vi "Process.vi"(8 "error in":errorcluster, 11 "Example Instrument":refnum<class "Instrument.LN2.lvclass">) -> (0 "error out":errorcluster, 3 "Example Instrument out":refnum<class "Instrument.LN2.lvclass">)   [LabVIEW 2019, in "Instrument.LN2.lvclass"]
doc: "---------------------------------------------------------------\nJKI State Machine Objects™\nhttp://jki.net/state-machine-objects/\nCopyright (C) 2005-2015, JKI <info@jki.net>\nALL RIGHTS RESERVED"
uses:
  Instrument.LN2.lvclass
  C:/Program Files (x86)/National Instruments/LabVIEW 2019/vi.lib/JKI/JKI SMO/SMO/SMO.lvclass
  C:/Program Files (x86)/National Instruments/LabVIEW 2019/user.lib/LevyLab/Instrument Framework/SMOs/Instrument/Instrument.lvclass
  Typedefs/PrivateEvents--Instrument.MessageToProcess.ctl
  <userlib>/LevyLab/Instrument Framework/SMOs/RemoteControl/Typedefs/Message--Cluster.ctl
  Instrument.LN2.lvclass/Instrument.LN2.ctl
  <vilib>/JKI/JKI SMO/SMO/SMO.lvclass/SMO.ctl
  Typedefs/Instrument.LN2.getAll--Cluster.ctl
  <vilib>/JKI/JKI SMO/SMO/Private/ReftoDVR--SMO.vi
  <userlib>/LevyLab/Instrument Framework/Instrument Types/VSource/Instrument.VSource.lvclass
  <vilib>/JKI/JKI SMO/SMO/SMO.lvclass
  <userlib>/LevyLab/Instrument Framework/SMOs/Instrument/Instrument.lvclass
  <userlib>/LevyLab/Instrument Framework/SMOs/RemoteControl/RemoteControl.lvclass
panel:
  # "LN2 process:\ntalks to hw"
  # "For instructions on how to use the JKI State Machine Objects, examples and video tutorials, visit:\nhttp://jki.net/state-machine-objects/\n\nJKI State Machine Objects™\nhttp://jki.net/state-machine-objects/\nCopyright (C) 2005-2015, JKI <info@jki.net>\nALL RIGHTS RESERVED"
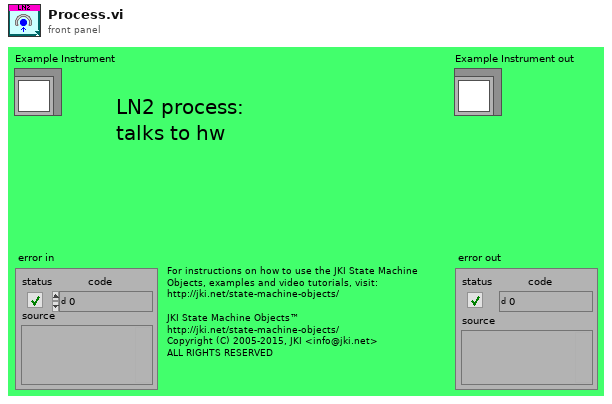
[diagram p1: front panel]
types:
  T1 = enum32{"invalid app kind", "Development System", "Run Time System", "Student Edition", "Embedded LabVIEW", "Evaluation", "Custom"}
  T2 = enum32{"Invalid", "Standard", "Closed", "Hidden", "Minimized", "Maximized"}
  T3 = enum32{"Bad", "Idle", "Run top level", "Running"}
  T4 = typedef "Instrument.LN2.lvclass/Instrument.LN2.getAll--Cluster.ctl" = cluster{"Net Weight(lbs)":dbl, "Level":dbl, "Status":string}
  T5 = typedef "RemoteControl.lvclass/Message--Cluster.ctl" = cluster{"Command":string, "Data":variant, "ID":string}
  T6 = typedef "Instrument.LN2.lvclass/PrivateEvents--Instrument.MessageToProcess.ctl" = cluster{"Message":T5}
  T7 = cluster{"Core":cluster{"Current VI Reference":refnum<vi>, "Close Panel on Exit?":bool, "Last Error":cluster{"error":errorcluster, "previous state":string, "remaining states":string}, "Shutdown?":bool}, "SelfRef":refnum<class "Instrument.LN2.lvclass">, "MessageToProcess":T6}
  T8 = cluster{"Current VI Reference":refnum<vi>, "Close Panel on Exit?":bool, "Last Error":cluster{"error":errorcluster, "previous state":string, "remaining states":string}, "Shutdown?":bool}
  T9 = typedef "SMO.lvclass/Protected Events.ctl" = cluster{"StopProcesses":refnum<user-event>, "AbortProcesses":refnum<user-event>, "Config Changed":refnum<user-event>, "Dependency":refnum<user-event>}
  T10 = typedef "Instrument.LN2.lvclass/PrivateEvents--Cluster.ctl" = cluster{"MessageToProcess":refnum<user-event>}
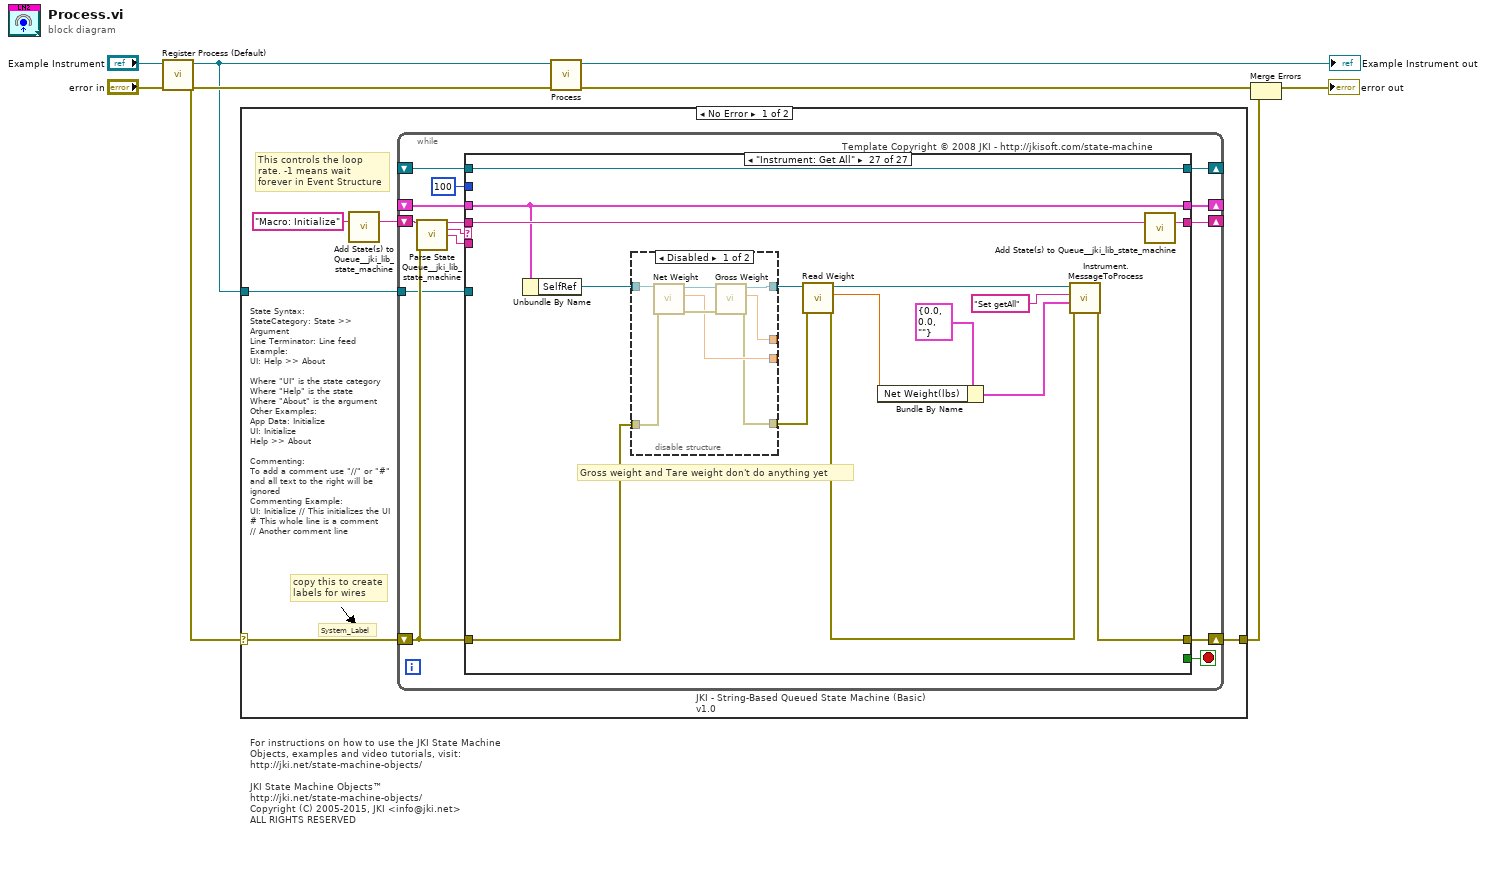
[diagram p0: block diagram]
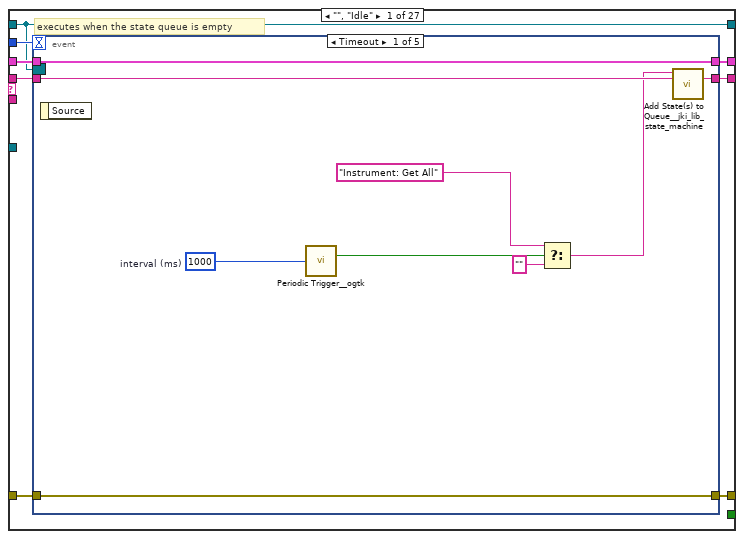
[diagram p2: hidden frame]
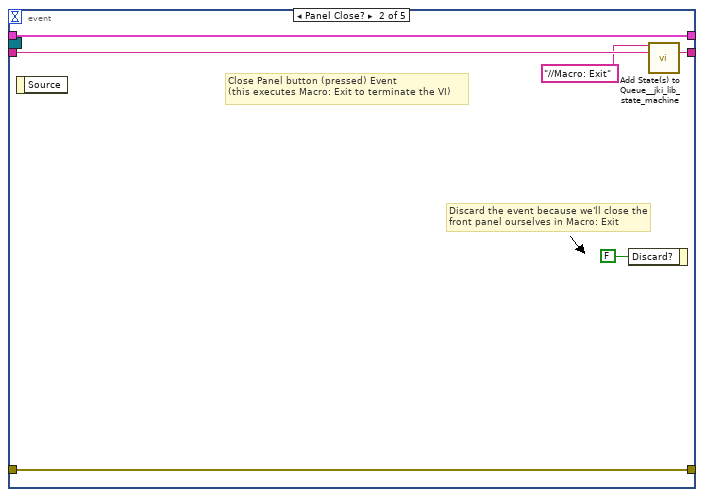
[diagram p3: hidden frame]
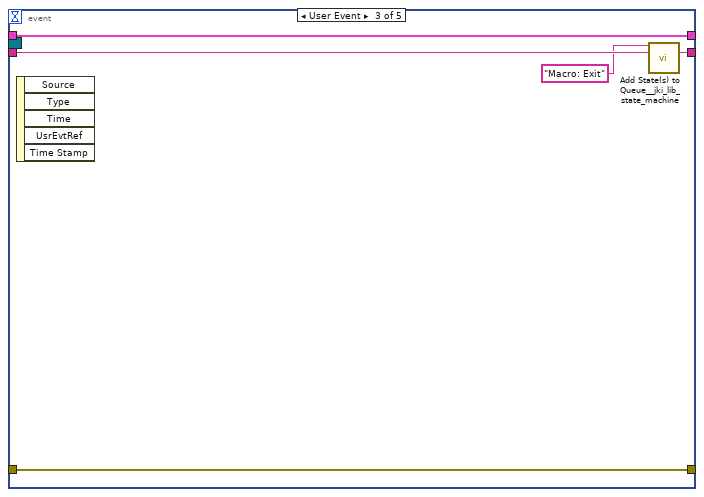
[diagram p4: hidden frame]
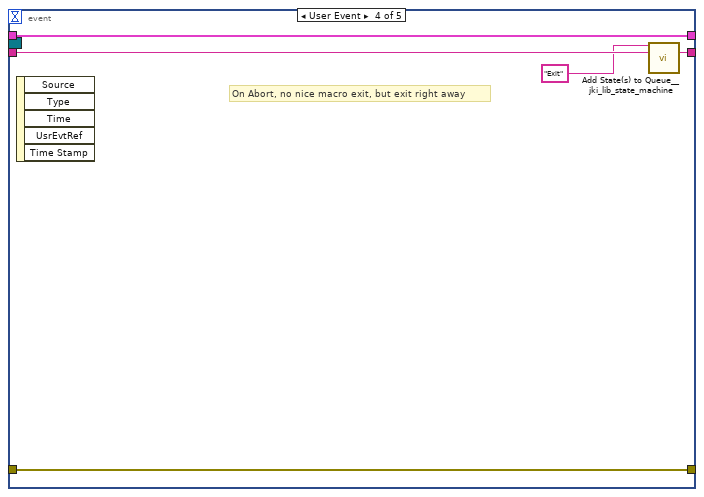
[diagram p5: hidden frame]
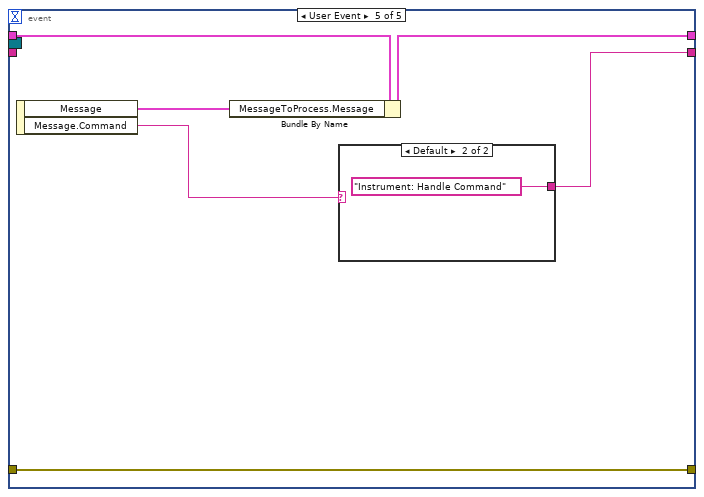
[diagram p6: hidden frame]
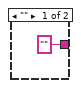
[diagram p7: hidden frame]
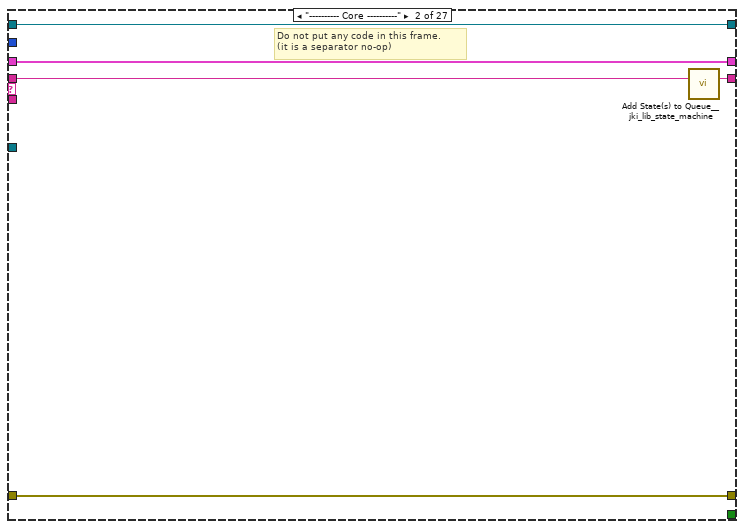
[diagram p8: hidden frame]
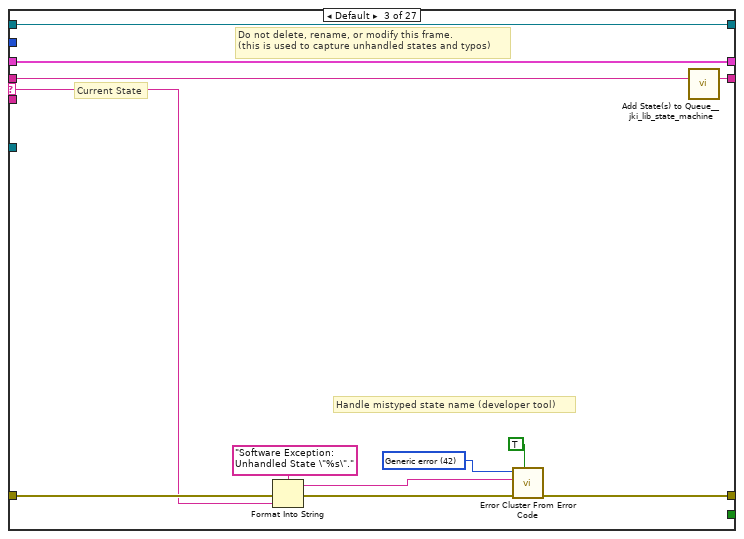
[diagram p9: hidden frame]
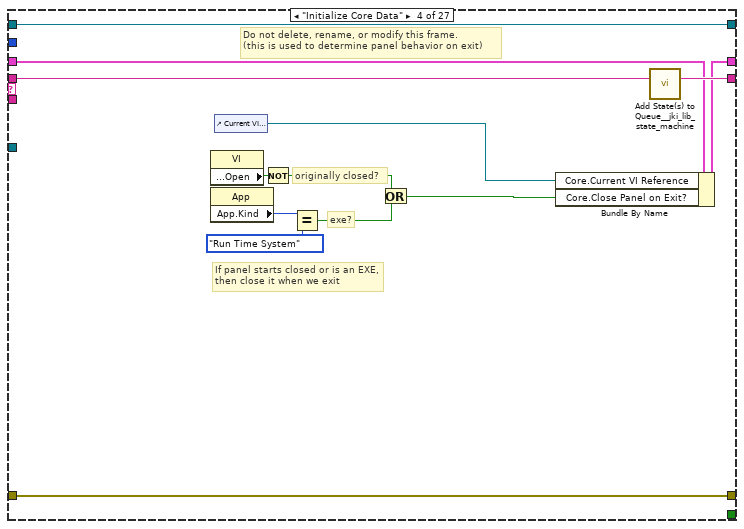
[diagram p10: hidden frame]
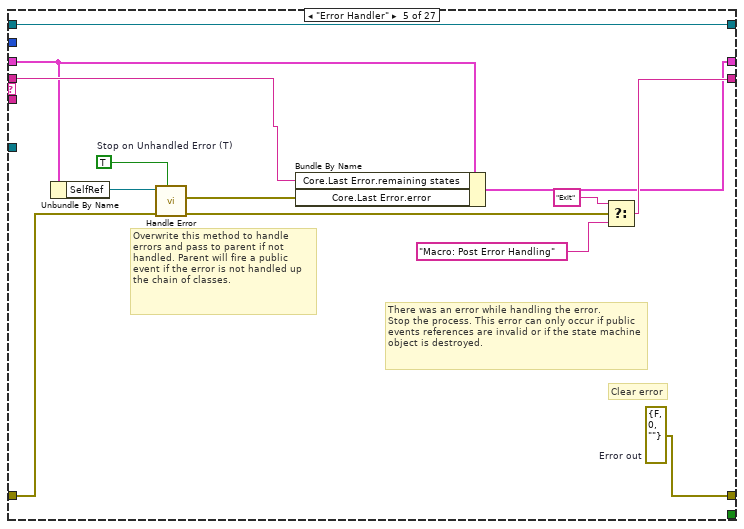
[diagram p11: hidden frame]
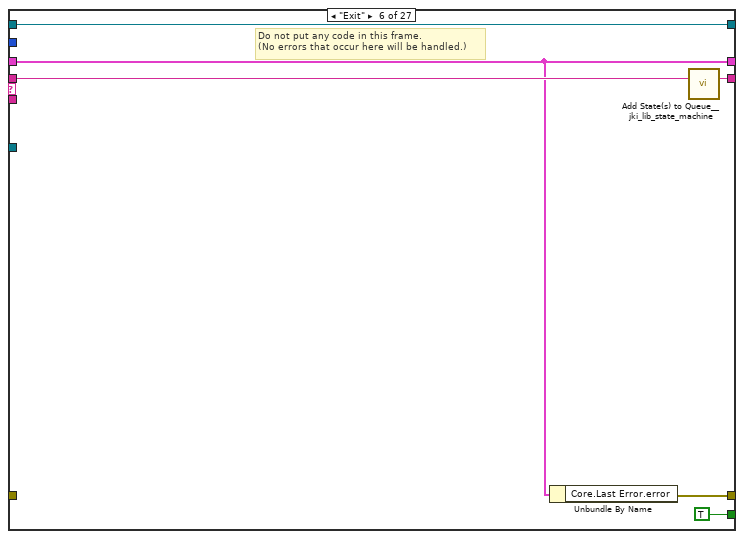
[diagram p12: hidden frame]
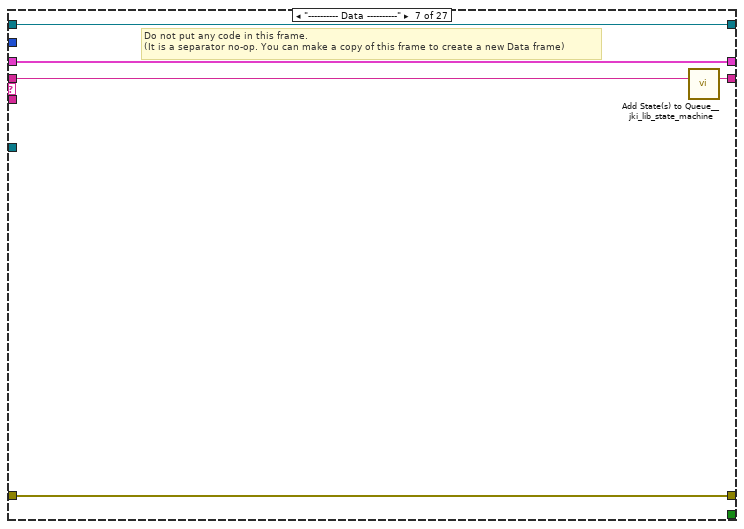
[diagram p13: hidden frame]
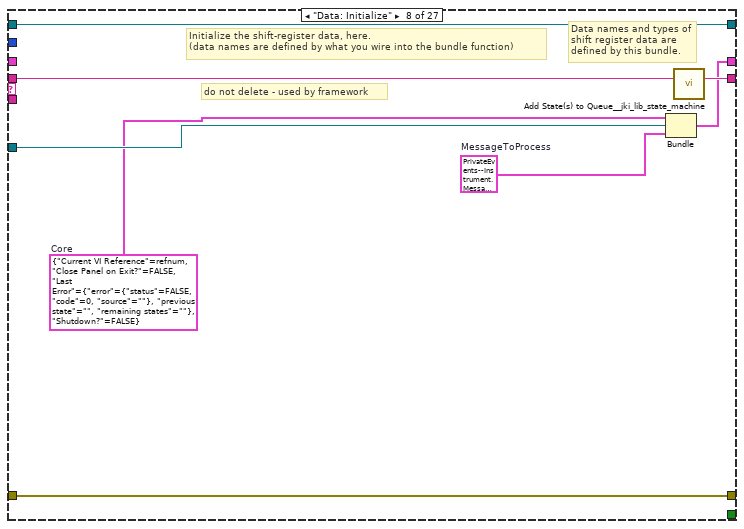
[diagram p14: hidden frame]
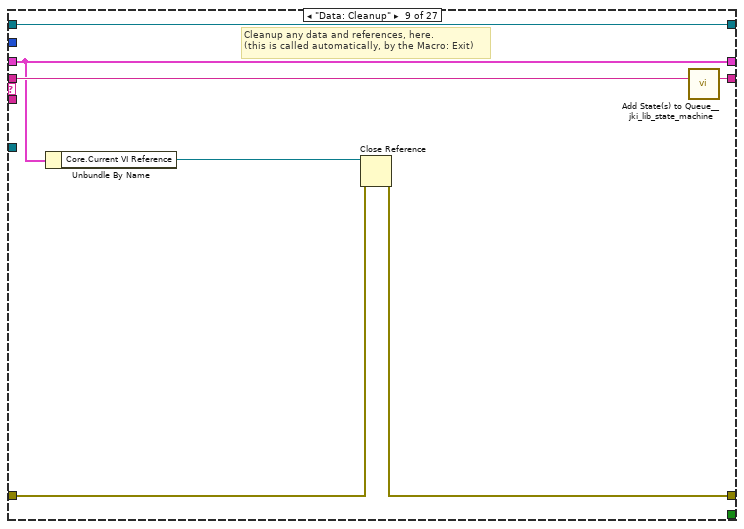
[diagram p15: hidden frame]
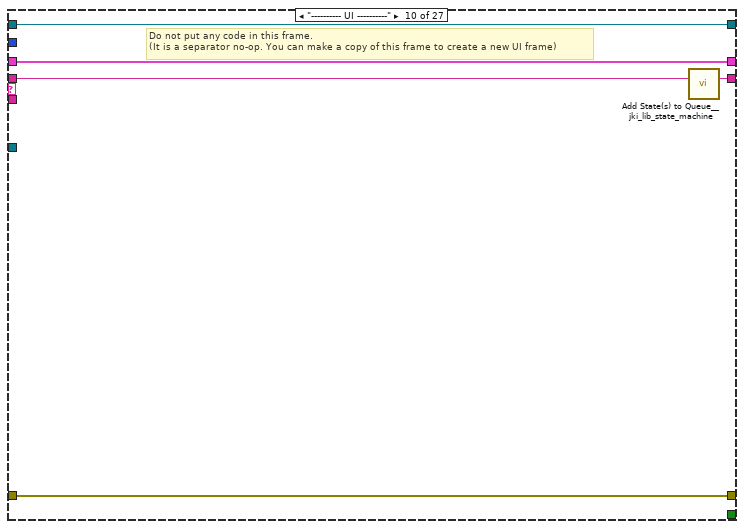
[diagram p16: hidden frame]
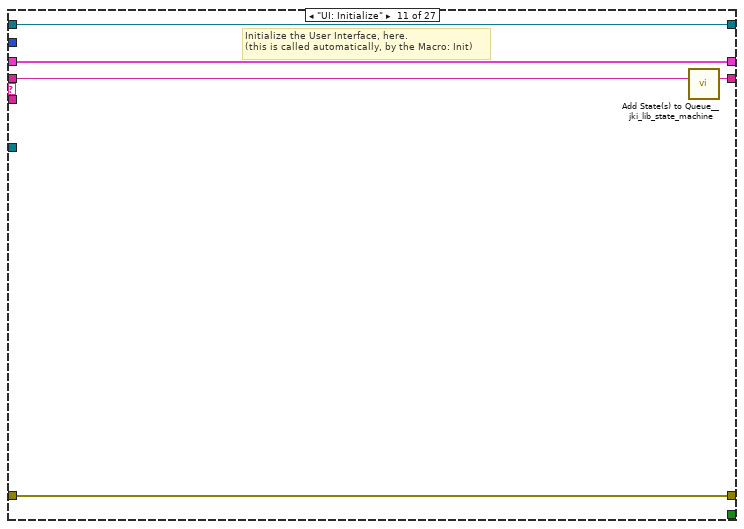
[diagram p17: hidden frame]
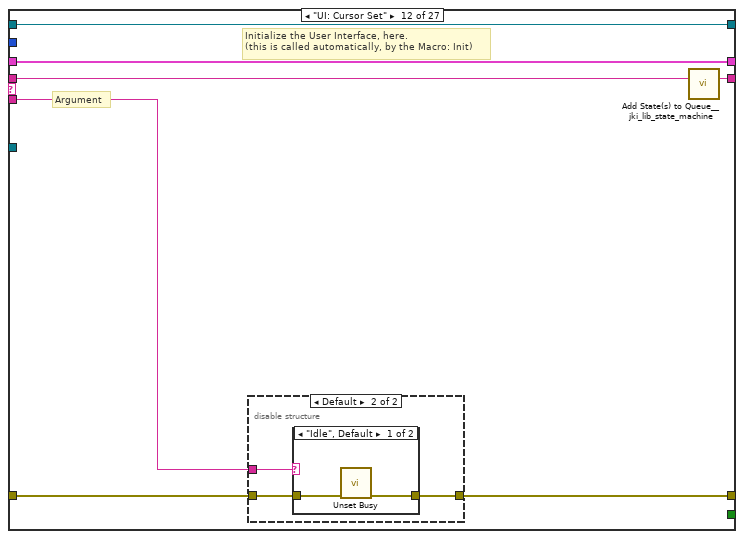
[diagram p18: hidden frame]
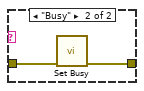
[diagram p20: hidden frame]
diagram:
  # "For instructions on how to use the JKI State Machine Objects, examples and video tutorials, visit:\nhttp://jki.net/state-machine-objects/\n\nJKI State Machine Objects™\nhttp://jki.net/state-machine-objects/\nCopyright (C) 2005-2015, JKI <info@jki.net>\nALL RIGHTS RESERVED"
  n1 = call <vilib>:"Register Process (Default).vi"("error in (no error)"="error in", "SMO"="Example Instrument") -> ("error out"=w5:errorcluster, "SelfRef"=w4:refnum<class "Instrument.LN2.lvclass">)  [unwired: 8 in]
  n2 = case shown="No Error" w5 {
    selector: w5 -> [w10 w357]
    tunnel: w4 -> [w11 _]
    tunnel: [w9 w357] -> w1
    frame No Error {
      # "State Syntax:\nStateCategory: State >> Argument\nLine Terminator: Line feed\nExample:\nUI: Help >> About\n\nWhere \"UI\" is the state category\nWhere \"Help\" is the state\nWhere \"About\" is the argument\nOther Examples:\nApp Data: Initialize\nUI: Initialize\nHelp >> About\n\nCommenting:\nTo add a comment use \"//\" or \"#\" and all text to the right will be ignored\nCommenting Example:\nUI: Initialize // This initializes the UI\n# This whole line is a comment\n// Another comment line"
      # "copy this to create labels for wires"
      # "This controls the loop rate. -1 means wait forever in Event Structure"
      # "System_Label"
      n3 = call <vilib>:"Add State(s) to Queue__jki_lib_state_machine.vi"("State(s) in (\"\")"="Macro: Initialize") -> ("States Out"=w13:string)  [unwired: 14 in]
      n4 = while "JKI - String-Based Queued State Machine (Basic) v1.0" {
        shift-right: [w21] -> _
        shift-left: _ -> [w20]
        shift-right: [w14] -> w9
        shift-left: w10 -> [w18]
        shift-right: [w23] -> _
        shift-left: w13 -> [w24]
        tunnel: w11 -> [w17]
        shift-right: [w16] -> _
        shift-left: _ -> [w15]
        stop <- w22 stop-if-true
        # "Template Copyright © 2008 JKI - http://jkisoft.com/state-machine"
        n5 = call <vilib>:"Parse State Queue__jki_lib_state_machine.vi"("State Queue"=w24, "Error In (no error)"=w18) -> ("Remaining States"=w26:string, "Current State"=w27:string, "Arguments"=w25:string)  [unwired: 11 in]
        n6 = case shown="\"Instrument: Get All\"" w27 {
          selector: w27 -> [_ _ w75 _ _ _ _ _ _ _ _ _ _ _ _ _ _ _ _ _ _ _ _ _ _ _ _]
          tunnel: w26 -> [w35 w73 w79 w98 w103 w117 w122 w130 w137 w142 w147 w154 w170 w202 w225 w246 w249 w267 w278 w283 w294 w300 w305 w310 w322 w331 w346]
          tunnel: w25 -> [_ _ _ _ _ _ _ _ _ _ _ w148 w164 _ _ _ _ _ _ _ _ _ _ _ _ _ _]
          tunnel: w20 -> [w33 w70 w77 w89 w101 w113 w119 _ w132 w139 w145 w152 w166 w199 w222 w227 w251 w264 w275 w280 w286 w298 w303 w306 w316 w327 w343]
          tunnel: w18 -> [w31 w71 w80 w95 w104 _ w120 w124 w134 w140 w144 w150 w168 w200 w205 w230 w248 w265 w270 w281 w290 w296 w301 w308 w314 w323 w334]
          tunnel: [w34 w72 w78 w97 w102 w116 w121 w129 w136 w141 w146 w153 w169 w201 w224 w245 w247 w266 w277 w282 w293 w299 w304 w309 w321 w330 w345] -> w23
          tunnel: [_ _ _ _ _ TRUE _ _ _ _ _ _ _ _ _ _ _ _ _ _ _ _ _ _ _ _ _] -> w22
          tunnel: [w30 w70 w77 w96 w100 w113 w119 w128 w132 w139 w145 w152 w166 w199 w222 w227 w250 w264 w275 w280 w286 w298 w303 w306 w317 w328 w343] -> w21
          tunnel: 100 ("Timeout") -> [w29 _ _ _ _ _ _ _ _ _ _ _ _ _ _ _ _ _ _ _ _ _ _ _ _ _ _]
          tunnel: w17 -> [_ _ _ _ _ _ _ w125 _ _ _ _ _ _ w213 w226 _ _ _ _ _ _ _ _ _ _ _]
          tunnel: [w28 w69 w74 w86 w111 w114 w118 w127 w131 w138 w143 w151 w163 w198 w223 w240 w258 w263 w276 w279 w292 w297 w302 w307 w320 w329 w344] -> w16
          tunnel: w15 -> [w28 w69 w74 w86 w111 w114 w118 w127 w131 w138 w143 w151 w163 w198 w223 w240 w258 w263 w276 w279 _ w297 w302 w307 w320 w329 w344]
          tunnel: [w32 w71 w81 w95 w99 w112 w120 w124 w133 w140 w144 w149 w167 w200 w204 w229 w248 w265 w269 w281 w289 w296 w301 w308 w315 w324 w336] -> w14
          frame "", "Idle" {
            # "executes when the state queue is empty"
            n7 = event shown="[0] Timeout" {
              selector: w28 -> [_ _ _ _ _]
              dyn-events: _ -> [_ _ _ _ _]
              timeout: w29 -> [_ _ _ _ _]
              tunnel: w35 -> [w44 w50 w55 w60 _]
              tunnel: [w43 w49 w54 w59 w62] -> w34
              tunnel: w33 -> [w41 w47 w52 w57 w66]
              tunnel: [w42 w48 w53 w58 w61] -> w32
              tunnel: w31 -> [w42 w48 w53 w58 w61]
              tunnel: [w41 w47 w52 w57 w65] -> w30
              event Timeout {
                w38 = u32 1000  # interval (ms)
                n8 = event-data() -> ()  [unwired: 1 in, 1 out]
                n9 = call <userlib>:"Periodic Trigger__ogtk.vi"("time (ms)"=w38) -> ("Triggered"=w40:bool)  [unwired: 12 in, 2 out]
                n10 = Select(t="Instrument: Get All" ("State(s) in Front (\"\")"), s=w40, f="") -> (s? t:f=w36:string)
                n11 = call <vilib>:"Add State(s) to Queue__jki_lib_state_machine.vi"("State(s) in Front (\"\")"=w36, "State(s) in (\"\")"=w44) -> ("States Out"=w43:string)  [unwired: 13 in]
              }
              event Panel Close? {
                # "Discard the event because we'll close the front panel ourselves in Macro: Exit"
                # "Close Panel button (pressed) Event\n(this executes Macro: Exit to terminate the VI)"
                n12 = event-data() -> ()  [unwired: 1 in, 1 out]
                n13 = event-data("Discard?"=FALSE) -> ()  [unwired: 1 in, 1 out]
                n14 = call <vilib>:"Add State(s) to Queue__jki_lib_state_machine.vi"("State(s) in Front (\"\")"="//Macro: Exit", "State(s) in (\"\")"=w50) -> ("States Out"=w49:string)  [unwired: 13 in]
              }
              event User Event {
                n15 = event-data() -> ()  [unwired: 1 in, 5 out]
                n16 = call <vilib>:"Add State(s) to Queue__jki_lib_state_machine.vi"("State(s) in Front (\"\")"="Macro: Exit", "State(s) in (\"\")"=w55) -> ("States Out"=w54:string)  [unwired: 13 in]
              }
              event User Event {
                # "On Abort, no nice macro exit, but exit right away"
                n17 = event-data() -> ()  [unwired: 1 in, 5 out]
                n18 = call <vilib>:"Add State(s) to Queue__jki_lib_state_machine.vi"("State(s) in Front (\"\")"="Exit", "State(s) in (\"\")"=w60) -> ("States Out"=w59:string)  [unwired: 13 in]
              }
              event User Event {
                n19 = event-data() -> ("Message"=w64:T5, "Message.Command"=w63:string)  [unwired: 1 in]
                n20 = Bundle By Name(cluster=w66, "MessageToProcess.Message"=w64) -> (w65:T7)
                n21 = case shown="Default" w63 {
                  tunnel: ["" ("States Out") "Instrument: Handle Command" ("States Out")] -> w62
                  frame "" {
                  }
                  frame Default {
                  }
                }
              }
            }
          }
          frame "---------- Core ----------" {
            # "Do not put any code in this frame.\n(it is a separator no-op)"
            n22 = call <vilib>:"Add State(s) to Queue__jki_lib_state_machine.vi"("State(s) in (\"\")"=w73) -> ("States Out"=w72:string)  [unwired: 14 in]
          }
          frame Default {
            w84 = 42 items=["No error", "Argument error", "Memory is full", "Out of zone", "End of file", "File already open", "Generic file I/O error", "File not found", "File permission error", "Disk is full", "Duplicate path", "Too many files open", "System feature not enabled", "Resource file not found", "Cannot add resource", "Resource not found", "Image not found", "Image memory error", "Pen does not exist", "Config type invalid", "Config token not found", "Config parse error", "Config memory error", "Bad external code format", "Bad external code offset", "External code not present", "Null window", "Destroy window error", "Null menu", "Print aborted", "Bad print record", "Print driver error", "Windows error during printing", "Memory error during printing", "Print dialog error", "Generic print error", "Invalid device refnum", "Device not found", "Device parameter error", "Device unit error", "Cannot open device", "Device call aborted", "Generic error", "Cancelled by user", "Object ID too low", "Object ID too high", "Object not in heap", "Unknown heap", "Unknown object (invalid DefProc)", "Unknown object (DefProc not in table)", "Message out of range", "Invalid (null) method", "Unknown message", "Manager call not supported", "Bad address", "Network operation in progress", "Network operation timed out", "Connection is busy", "Network attribute not supported", "Network error", "Address in use", "System out of memory", "Connection aborted", "Connection refused", "Not connected", "Already connected", "Connection closed", "Initialization error (interapplication manager)", "Bad occurrence", "Wait on unbound occurrence handler", "Occurrence queue overflow", "Datalog type conflict", "Unused", "Unrecognized type (interapplication manager)", "Memory corrupt", "Failed to make temporary DLL", "Old CIN version", "Drag socket not found", "Failed to load drop-object", "Failed to register OLE object", "Failed to release OLE object", "Format specifier type mismatch", "Unknown format specifier", "Too few format specifiers", "Too many format specifiers", "Scan failed", "Newer CIN version", "Error converting to variant", "Runtime menu error", "Password tampered", "Variant attribute not found", "Incompatible variant data type", "Event data is not available", "Event Store is not present", "Occurrence is not found", "Event Queue is not created", "Event info is not available", "Refnum passed is NULL", "Error retrieving Class GUID", "Error retrieving CoClass GUID", "Error retrieving TypeLib GUID.", "Bad built application magic bytes.", "Specific driver is different from the specific driver associated with the Logical Name.", "There is no session opened to the class driver.", "Max Error", "MAX - Error with config objects", "MAX - Error loading configuration", "MAX - Group not supported"]
            # "Current State"
            # "Do not delete, rename, or modify this frame.\n(this is used to capture unhandled states and typos)"
            # "Handle mistyped state name (developer tool)"
            n23 = Format Into String(format string="Software Exception: Unhandled State \"%s\"." ("message"), error in=w80, w75) -> (resulting string=w83:string, error out=w82:errorcluster)  [unwired: 1 in]
            n24 = call <vilib>:"Error Cluster From Error Code.vi"("show call chain? (False)"=TRUE, "error in (no error)"=w82, "error message (\"\")"=w83, "error code (0)"=w84) -> ("error out"=w81:errorcluster)  [unwired: 5 in]
            n25 = call <vilib>:"Add State(s) to Queue__jki_lib_state_machine.vi"("State(s) in (\"\")"=w79) -> ("States Out"=w78:string)  [unwired: 14 in]
          }
          frame "Initialize Core Data" {
            # "Do not delete, rename, or modify this frame.\n(this is used to determine panel behavior on exit)"
            # "originally closed?"
            # "exe?"
            # "If panel starts closed or is an EXE, then close it when we exit"
            n26 = property class="VI"() -> ("Front Panel.Open"=w94:bool)  [unwired: 2 in, 2 out]
            n27 = property class="App"() -> ("App.Kind"=w93:T1)  [unwired: 2 in, 2 out]
            n28 = control-ref of="Current VI Reference"() -> (w87:refnum<vi>)
            n29 = Not(x=w94) -> (.not. x?=w91:bool)
            n30 = Equal?(x=w93, y=T1."Run Time System" ("Application:Kind")) -> (x = y?=w90:bool)
            n31 = Or(x=w91, y=w90) -> (x .or. y?=w88:bool)
            n32 = Bundle By Name(cluster=w89, "Core.Current VI Reference"=w87, "Core.Close Panel on Exit?"=w88) -> (w96:T7)
            n33 = call <vilib>:"Add State(s) to Queue__jki_lib_state_machine.vi"("State(s) in (\"\")"=w98) -> ("States Out"=w97:string)  [unwired: 14 in]
          }
          frame "Error Handler" {
            w99 = errorcluster {"status"=FALSE, "code"=0, "source"=""}  # Error out
            w109 = TRUE  # Stop on Unhandled Error (T)
            # "Clear error"
            # "There was an error while handling the error.\nStop the process. This error can only occur if public events references are invalid or if the state machine object is destroyed."
            # "Overwrite this method to handle errors and pass to parent if not handled. Parent will fire a public event if the error is not handled up the chain of classes."
            n34 = Unbundle By Name(w101) -> ("SelfRef"=w106:refnum<class "Instrument.LN2.lvclass">)
            n35 = call-dynamic "Handle Error.vi"("Stop on Unhandled Error (T)"=w109, "error in"=w104, "SMO"=w106) -> ("handling error"=w107:errorcluster, "Unhandled error"=w108:errorcluster)  [unwired: 6 in, 1 out]
            n36 = Bundle By Name(cluster=w101, "Core.Last Error.remaining states"=w103, "Core.Last Error.error"=w108) -> (w100:T7)
            n37 = Select(t="Exit", s=w107, f="Macro: Post Error Handling" ("State")) -> (s? t:f=w102:string)
          }
          frame "Exit" {
            # "Do not put any code in this frame.\n(No errors that occur here will be handled.)"
            n38 = Unbundle By Name(w113) -> ("Core.Last Error.error"=w112:errorcluster)
            n39 = call <vilib>:"Add State(s) to Queue__jki_lib_state_machine.vi"("State(s) in (\"\")"=w117) -> ("States Out"=w116:string)  [unwired: 14 in]
          }
          frame "---------- Data ----------" {
            # "Do not put any code in this frame.\n(It is a separator no-op. You can make a copy of this frame to create a new Data frame)"
            n40 = call <vilib>:"Add State(s) to Queue__jki_lib_state_machine.vi"("State(s) in (\"\")"=w122) -> ("States Out"=w121:string)  [unwired: 14 in]
          }
          frame "Data: Initialize" {
            w123 = T8 {"Current VI Reference"=refnum, "Close Panel on Exit?"=FALSE, "Last Error"={"error"={"status"=FALSE, "code"=0, "source"=""}, "previous state"="", "remaining states"=""}, "Shutdown?"=FALSE}  # Core
            w126 = T6 {"Message"={"Command"="", "Data"=variant(string ""), "ID"=""}}  # MessageToProcess
            # "do not delete - used by framework"
            # "Data names and types of shift register data are defined by this bundle."
            # "Initialize the shift-register data, here.\n(data names are defined by what you wire into the bundle function)"
            n41 = Bundle("Core"=w123, "SelfRef"=w125, "MessageToProcess"=w126) -> (w128:T7)  [unwired: 1 in]
            n42 = call <vilib>:"Add State(s) to Queue__jki_lib_state_machine.vi"("State(s) in (\"\")"=w130) -> ("States Out"=w129:string)  [unwired: 14 in]
          }
          frame "Data: Cleanup" {
            # "Cleanup any data and references, here.\n(this is called automatically, by the Macro: Exit)"
            n43 = Unbundle By Name(w132) -> ("Core.Current VI Reference"=w135:refnum<vi>)
            n44 = Close Reference(reference=w135, error in (no error)=w134) -> (error out=w133:errorcluster)
            n45 = call <vilib>:"Add State(s) to Queue__jki_lib_state_machine.vi"("State(s) in (\"\")"=w137) -> ("States Out"=w136:string)  [unwired: 14 in]
          }
          frame "---------- UI ----------" {
            # "Do not put any code in this frame.\n(It is a separator no-op. You can make a copy of this frame to create a new UI frame)"
            n46 = call <vilib>:"Add State(s) to Queue__jki_lib_state_machine.vi"("State(s) in (\"\")"=w142) -> ("States Out"=w141:string)  [unwired: 14 in]
          }
          frame "UI: Initialize" {
            # "Initialize the User Interface, here.\n(this is called automatically, by the Macro: Init)"
            n47 = call <vilib>:"Add State(s) to Queue__jki_lib_state_machine.vi"("State(s) in (\"\")"=w147) -> ("States Out"=w146:string)  [unwired: 14 in]
          }
          frame "UI: Cursor Set" {
            # "Argument"
            # "Initialize the User Interface, here.\n(this is called automatically, by the Macro: Init)"
            n48 = disable-structure shown="Default" {
              disable-tunnel: w150 -> [w155 w158]
              disable-tunnel: [w155 w157] -> w149
              disable-tunnel: w148 -> [_ w156]
              frame condition #0 {
              }
              frame condition #1 (active) {
                n49 = case shown="\"Idle\", Default" w156 {
                  tunnel: w158 -> [w160 w162]
                  tunnel: [w159 w161] -> w157
                  frame "Idle", Default {
                    n50 = call <vilib>:"Unset Busy.vi"("error in (no error)"=w160) -> ("error out"=w159:errorcluster)  [unwired: 10 in]
                  }
                  frame "Busy" {
                    n51 = call <vilib>:"Set Busy.vi"("error in (no error)"=w162) -> ("error out"=w161:errorcluster)  [unwired: 9 in, 1 out]
                  }
                }
              }
            }
            n52 = call <vilib>:"Add State(s) to Queue__jki_lib_state_machine.vi"("State(s) in (\"\")"=w154) -> ("States Out"=w153:string)  [unwired: 14 in]
          }
          frame "UI: Front Panel State" {
            # "Argument"
            # "Set Front Panel Open or Closed\n(Usage: \"UI: Front Panel State >> Open|Close\")"
            n53 = Unbundle By Name(w166) -> ("Core.Current VI Reference"=w165:refnum<vi>)
            n54 = disable-structure shown="Default" {
              disable-tunnel: w168 -> [w174 w197]
              disable-tunnel: [w173 w197] -> w167
              disable-tunnel: w165 -> [w172 _]
              disable-tunnel: w164 -> [w171 _]
              frame condition #0 (active) {
                n55 = case shown="\"Open\", Default" w171 {
                  tunnel: w174 -> [w178 w191]
                  tunnel: [w180 w192] -> w173
                  tunnel: w172 -> [w179 w189]
                  frame "Open", Default {
                    n56 = property class="VI"(reference=w179, error in=w178) -> (reference out=w176:refnum<vi>, error out=w177:errorcluster, "FP.State"=w175:T2)
                    n57 = case shown="\"Closed\"" w175 {
                      tunnel: [w183 w186] -> w180
                      tunnel: w177 -> [w182 w186]
                      tunnel: w176 -> [w181 _]
                      frame "Closed" {
                        n58 = invoke class="VI" method="FP.Open"(reference=w181, error in=w182, "Activate"=TRUE, "State"=T2."Standard") -> (error out=w183:errorcluster)  [unwired: 1 in, 4 out]
                      }
                      frame Default {
                      }
                    }
                  }
                  frame "Close" {
                    n59 = property class="VI"(reference=w189, error in=w191) -> (reference out=w188:refnum<vi>, error out=w190:errorcluster, "FP.State"=w187:T2)
                    n60 = case shown="Default" w187 {
                      tunnel: [w193 w196] -> w192
                      tunnel: w190 -> [w193 w195]
                      tunnel: w188 -> [_ w194]
                      frame "Invalid", "Closed" {
                      }
                      frame Default {
                        n61 = invoke class="VI" method="FP.Close"(reference=w194, error in=w195) -> (error out=w196:errorcluster)  [unwired: 1 in, 2 out]
                      }
                    }
                  }
                }
              }
              frame condition #1 {
              }
            }
            n62 = call <vilib>:"Add State(s) to Queue__jki_lib_state_machine.vi"("State(s) in (\"\")"=w170) -> ("States Out"=w169:string)  [unwired: 14 in]
          }
          frame "---------- Macro ----------" {
            # "Do not put any code in this frame.\n(It is a separator no-op. You can make a copy of this frame to create a new Macro frame)"
            n63 = call <vilib>:"Add State(s) to Queue__jki_lib_state_machine.vi"("State(s) in (\"\")"=w202) -> ("States Out"=w201:string)  [unwired: 14 in]
          }
          frame "Macro: Initialize" {
            w214 = "Process: Sync"
            # "Initialization Macro\n(This is called once, when the VI starts)"
            n64 = control-ref of="This VI"() -> (w216:refnum<vi>)
            n65 = property class="VI"(reference=w216) -> ("Exec.State"=w215:T3)  [unwired: 1 in, 2 out]
            n66 = call-dynamic "Read Debug Mode.vi"("error in (no error)"=w205, "Instrument in"=w213) -> ("error out"=w204:errorcluster, "Debug Mode?"=w206:bool)  [unwired: 7 in, 1 out]
            n67 = Equal?(x=w215, y=T3."Run top level") -> (x = y?=w220:bool)
            n68 = Select(t="Open", s=w206, f="Close") -> (s? t:f=w211:string)
            n69 = call <vilib>:"Build State String with Arguments__JKI_lib_State_Machine.vi"("Arguments (\"\")"=w211, "State"="UI: Front Panel State") -> ("State with Arguments"=w208:string)  [unwired: 4 in]
            n70 = Select(t=w214, s=w220, f="") -> ()  [unwired: 1 out]
            n71 = call <vilib>:"Add State(s) to Queue__jki_lib_state_machine.vi"("State(s) in Front (\"\")"="UI: Initialize\nInstrument: Open", "State(s) in (\"\")"=w208) -> ("States Out"=w203:string)  [unwired: 13 in]
            n72 = call <vilib>:"Add State(s) to Queue__jki_lib_state_machine.vi"("State(s) in Front (\"\")"="Data: Initialize\nInitialize Core Data\nEvents: Register", "State(s) in (\"\")"=w214, "State(s) at Back (\"\")"=w203) -> ("States Out"=w217:string)  [unwired: 12 in]
            n73 = call <vilib>:"Add State(s) to Queue__jki_lib_state_machine.vi"("State(s) in Front (\"\")"=w217, "State(s) in (\"\")"=w225) -> ("States Out"=w224:string)  [unwired: 13 in]
          }
          frame "Macro: Exit" {
            # "Exit Macro\n(This is called once, when the VI exits)"
            n74 = Unbundle By Name(w227) -> ("Core.Close Panel on Exit?"=w244:bool)
            n75 = call-dynamic "Read Debug Mode.vi"("error in (no error)"=w230, "Instrument in"=w226) -> ("error out"=w229:errorcluster, "Debug Mode?"=w228:bool)  [unwired: 7 in, 1 out]
            n76 = Select(t="Open", s=w228, f="Close") -> (s? t:f=w234:string)
            n77 = call <vilib>:"Build State String with Arguments__JKI_lib_State_Machine.vi"("Arguments (\"\")"=w234, "State"="UI: Front Panel State") -> ("State with Arguments"=w231:string)  [unwired: 4 in]
            n78 = Select(t=w231, s=w244, f="") -> (s? t:f=w242:string)
            n79 = call <vilib>:"Add State(s) to Queue__jki_lib_state_machine.vi"("State(s) in Front (\"\")"="Instrument: Close\nData: Cleanup\nEvents: Unregister", "State(s) in (\"\")"="Process: Sync", "State(s) at Back (\"\")"="Exit") -> ("States Out"=w237:string)  [unwired: 12 in]
            n80 = call <vilib>:"Add State(s) to Queue__jki_lib_state_machine.vi"("State(s) in (\"\")"=w242, "State(s) at Back (\"\")"=w237) -> ("States Out"=w241:string)  [unwired: 13 in]
            n81 = call <vilib>:"Add State(s) to Queue__jki_lib_state_machine.vi"("State(s) in Front (\"\")"=w241, "State(s) in (\"\")"=w246) -> ("States Out"=w245:string)  [unwired: 13 in]
          }
          frame "Macro: Post Error Handling" {
            # "Clear Last Error?"
            n82 = Unbundle By Name(w251) -> ("Core.Last Error.remaining states"=w256:string, "Core.Shutdown?"=w257:bool)
            n83 = Unbundle By Name(w251) -> ("Core.Last Error.error"=w253:errorcluster)
            n84 = case shown="False" FALSE {
              tunnel: w253 -> [w259 _]
              tunnel: [w259 _] -> w252
              frame False {
              }
              frame True {
              }
            }
            n85 = case shown="True" w257 {
              tunnel: w256 -> [w260 w262]
              tunnel: [w260 w261] -> w255
              frame False {
                # "These are the remaining states (at the moment the error occured). States can be altered according to business logic."
                # "NOT SHUTTING DOWN"
              }
              frame True {
                # "Developer can decide to alter the states but should be aware that during the shutdown process, there are certain states that must be run for the SMO to properly shut itself (and this process) down. As such, one can add states to perform additional clean-ups, but should append the remaining state to be executed."
                # "SHUTTING DOWN"
                n86 = call <vilib>:"Add State(s) to Queue__jki_lib_state_machine.vi"("State(s) in (\"\")"=w262) -> ("States Out"=w261:string)  [unwired: 14 in]
              }
            }
            n87 = Bundle By Name(cluster=w251, "Core.Last Error.error"=w252) -> (w250:T7)
            n88 = call <vilib>:"Add State(s) to Queue__jki_lib_state_machine.vi"("State(s) in Front (\"\")"=w255, "State(s) in (\"\")"=w249) -> ("States Out"=w247:string)  [unwired: 13 in]
          }
          frame "---------- Process ----------" {
            # "Template Separator\n(You can make a copy of, or modify, this frame)"
            n89 = call <vilib>:"Add State(s) to Queue__jki_lib_state_machine.vi"("State(s) in (\"\")"=w267) -> ("States Out"=w266:string)  [unwired: 14 in]
          }
          frame "Process: Sync" {
            n90 = Unbundle By Name(w275) -> ("SelfRef"=w271:refnum<class "Instrument.LN2.lvclass">)
            n91 = call <vilib>:"WaitOnProcessSync.vi"("error in (no error)"=w270, "SMO"=w271) -> ("error out"=w269:errorcluster, "Don't run?"=w274:bool)  [unwired: 7 in, 1 out]
            n92 = Select(t="Data: Cleanup\nEvents: Unregister\nExit", s=w274, f="") -> (s? t:f=w268:string)
            n93 = call <vilib>:"Add State(s) to Queue__jki_lib_state_machine.vi"("State(s) in Front (\"\")"=w268, "State(s) in (\"\")"=w278) -> ("States Out"=w277:string)  [unwired: 13 in]
          }
          frame "---------- Events ----------" {
            # "Template Separator\n(You can make a copy of, or modify, this frame)"
            n94 = call <vilib>:"Add State(s) to Queue__jki_lib_state_machine.vi"("State(s) in (\"\")"=w283) -> ("States Out"=w282:string)  [unwired: 14 in]
          }
          frame "Events: Register" {
            # "Expand to add\nmore events"
            n95 = Unbundle By Name(w286) -> ("SelfRef"=w285:refnum<class "Instrument.LN2.lvclass">)
            n96 = call <vilib>:"GetProtectedEvents.vi"("SMO"=w285) -> ("error out"=w287:errorcluster, "SMO Protected Events"=w291:T9)  [unwired: 8 in, 1 out]
            n97 = call "LN2.GetPrivateEvents.vi"("Instrument.LN2 in"=w285) -> ("PrivateEvents"=w284:T10)  [unwired: 8 in, 2 out]
            n98 = register-events(w291, w284) -> (reference out=w292:refnum<event-registration>, error out=w288:errorcluster)  [unwired: 2 in]
            n99 = Merge Errors(w290, w288, w287) -> (w289:errorcluster)
            n100 = call <vilib>:"Add State(s) to Queue__jki_lib_state_machine.vi"("State(s) in (\"\")"=w294) -> ("States Out"=w293:string)  [unwired: 14 in]
          }
          frame "Events: Unregister" {
            n101 = Unregister For Events(event registration refnum=w297, error in=w296) -> (error out=w295:errorcluster)
            n102 = call <vilib>:"Clear Errors.vi"("error in (no error)"=w295) -> ()  [unwired: 5 in, 2 out]
            n103 = call <vilib>:"Add State(s) to Queue__jki_lib_state_machine.vi"("State(s) in (\"\")"=w300) -> ("States Out"=w299:string)  [unwired: 14 in]
          }
          frame "---------- Instrument ----------" {
            n104 = call <vilib>:"Add State(s) to Queue__jki_lib_state_machine.vi"("State(s) in (\"\")"=w305) -> ("States Out"=w304:string)  [unwired: 14 in]
          }
          frame "Instrument: Handle Command" {
            n105 = Unbundle By Name(w306) -> ()  [unwired: 1 out]
            n106 = disable-structure shown="Enabled" {
              frame Disabled {
                n107 = call "Net Weight.vi"() -> ("error out"=w312:errorcluster, "Instrument.LN2 out"=w313:refnum<class "Instrument.LN2.lvclass">)  [unwired: 9 in, 1 out]
                n108 = call "Gross Weight.vi"("error in (no error)"=w312, "Instrument.LN2 in"=w313) -> ("Instrument.LN2 out"=w311:refnum<class "Instrument.LN2.lvclass">)  [unwired: 7 in, 2 out]
                n109 = call "Read Weight.vi"("Instrument.LN2 in"=w311) -> ()  [unwired: 8 in, 3 out]
                n110 = call <userlib>:"Instrument.MessageToProcess.vi"() -> ()  [unwired: 10 in, 2 out]
              }
              frame Enabled {
              }
            }
            n111 = call <vilib>:"Add State(s) to Queue__jki_lib_state_machine.vi"("State(s) in (\"\")"=w310) -> ("States Out"=w309:string)  [unwired: 14 in]
          }
          frame "Instrument: Open" {
            n112 = Unbundle By Name(w316) -> ("SelfRef"=w319:refnum<class "Instrument.LN2.lvclass">)
            n113 = call-dynamic "Open Hardware.vi"("error in (no error)"=w314, "Instrument.Template in"=w319) -> ("error out"=w315:errorcluster, "Instrument.Template out"=w318:refnum<class "Instrument.LN2.lvclass">)  [unwired: 8 in]
            n114 = Bundle By Name(cluster=w316, "SelfRef"=w318) -> (w317:T7)
            n115 = call <vilib>:"Add State(s) to Queue__jki_lib_state_machine.vi"("State(s) in (\"\")"=w322) -> ("States Out"=w321:string)  [unwired: 14 in]
          }
          frame "Instrument: Close" {
            n116 = Unbundle By Name(w327) -> ("SelfRef"=w326:refnum<class "Instrument.LN2.lvclass">)
            n117 = call-dynamic "Close Hardware.vi"("error in (no error)"=w323, "Instrument.Template in"=w326) -> ("error out"=w324:errorcluster, "Instrument.Template out"=w325:refnum<class "Instrument.LN2.lvclass">)  [unwired: 8 in]
            n118 = Bundle By Name(cluster=w327, "SelfRef"=w325) -> (w328:T7)
            n119 = call <vilib>:"Add State(s) to Queue__jki_lib_state_machine.vi"("State(s) in (\"\")"=w331) -> ("States Out"=w330:string)  [unwired: 14 in]
          }
          frame "Instrument: Get All" {
            # "Gross weight and Tare weight don't do anything yet"
            n120 = Unbundle By Name(w343) -> ("SelfRef"=w341:refnum<class "Instrument.LN2.lvclass">)
            n121 = disable-structure shown="Disabled" {
              disable-tunnel: [w352 w356] -> w342
              disable-tunnel: w341 -> [w351 w356]
              disable-tunnel: [w347 w355] -> w340
              disable-tunnel: [w350 _] -> _
              disable-tunnel: [w349 _] -> _
              disable-tunnel: w334 -> [w348 w355]
              frame Disabled {
                n122 = call "Net Weight.vi"("error in (no error)"=w348, "Instrument.LN2 in"=w351) -> ("error out"=w353:errorcluster, "Net Weight (kg)"=w350:dbl, "Instrument.LN2 out"=w354:refnum<class "Instrument.LN2.lvclass">)  [unwired: 7 in]
                n123 = call "Gross Weight.vi"("error in (no error)"=w353, "Instrument.LN2 in"=w354) -> ("error out"=w347:errorcluster, "Get Weight"=w349:dbl, "Instrument.LN2 out"=w352:refnum<class "Instrument.LN2.lvclass">)  [unwired: 7 in]
              }
              frame Enabled {
              }
            }
            n124 = call "Read Weight.vi"("error in (no error)"=w340, "Instrument.LN2 in"=w342) -> ("error out"=w333:errorcluster, "Weight"=w332:dbl, "Instrument.LN2 out"=w335:refnum<class "Instrument.LN2.lvclass">)  [unwired: 7 in]
            n125 = Bundle By Name(cluster=T4 {"Net Weight(lbs)"=0.0, "Level"=0.0, "Status"=""} ("getAll"), "Net Weight(lbs)"=w332) -> (w338:T4)
            n126 = call <userlib>:"Instrument.MessageToProcess.vi"("error in (no error)"=w333, "Data"=w338, "Command"="Set getAll", "Instrument"=w335) -> ("error out"=w336:errorcluster)  [unwired: 6 in, 1 out]
            n127 = call <vilib>:"Add State(s) to Queue__jki_lib_state_machine.vi"("State(s) in (\"\")"=w346) -> ("States Out"=w345:string)  [unwired: 14 in]
          }
        }
      }
    }
    frame Error {
    }
  }
  n128 = call-parent "Process.vi"("error in"=w5, "Instrument"=w4) -> ("error out"=w2:errorcluster, "Instrument out"=→"Example Instrument out":refnum<class "Instrument.LN2.lvclass">)  [unwired: 8 in]
  n129 = Merge Errors(w2, w1) -> (→"error out":errorcluster)
